vi "Memory.Pointer.Read Bytes.Safe.vi"(8 "error in (no error)":errorcluster, 11 "Pointer in":refnum<class "Memory.Pointer.lvclass">) -> (0 "error out":errorcluster, 2 "buffer":u8[](array[numeric]) format="%02x", 3 "Pointer out":refnum<class "Memory.Pointer.lvclass">)   [LabVIEW 2016, in "LabVIEW Memory Manager.lvlib" / "Memory.Pointer.lvclass"]
uses:
  Memory.Pointer.lvclass
  Memory.Pointer.lvclass/Memory.Pointer.ctl
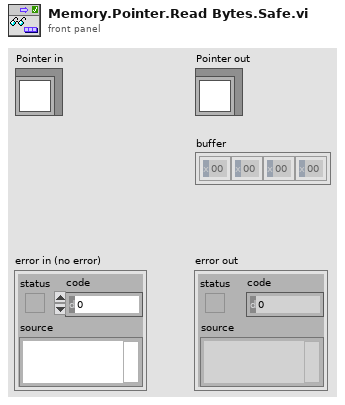
[diagram p1: front panel]
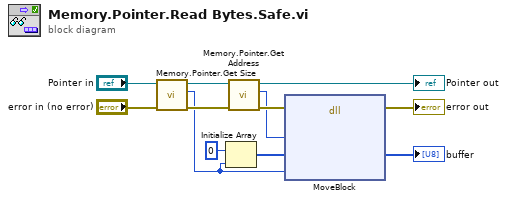
[diagram p0: block diagram]
diagram:
  n1 = call "Memory.Pointer.Get Size.vi"("error in (no error)"="error in (no error)", "Pointer in"="Pointer in") -> ("error out"=w12:errorcluster, "size"=w1:u64, "Pointer out"=w11:refnum<class "Memory.Pointer.lvclass">)  [unwired: 7 in]
  n2 = Initialize Array(u8 0 ("element"), w1) -> (w2:u8[])
  n3 = call "Memory.Pointer.Get Address.vi"("error in (no error)"=w12, "Pointer in"=w11) -> ("error out"=w10:errorcluster, "address"=w9:u64, "Pointer out"=→"Pointer out":refnum<class "Memory.Pointer.lvclass">)  [unwired: 7 in]
  n4 = dll-call lib="LabVIEW" fn="MoveBlock"(error in=w10, "src pointer"=w9, "dst pointer"=w2, "size"=w1) -> (error out=→"error out":errorcluster, "dst pointer"=→"buffer":u8[])  [unwired: 5 in, 1 out]
